vi "averaged_asap_signals.vi"(8 "error in":errorcluster, 10 "Averaging time (ms)":u32=1000, 11 "Settling time (ms)":u32=1000) -> (0 "error out":errorcluster, 1 "ASAP diagnostics":cluster{"Valid position":bool, "Message":string}, 2 "Poses":sgl[][](array[numeric]), 3 "Demodulated averaged":sgl[][](array[numeric]))   [LabVIEW 2013]
doc: "I. Description:\nThis example demonstrates how to acquire a continuous amount of data (Waveform) using the DAQ device's internal clock.\n\nII. Instructions for Running:\n1. Create an analog input voltage channel.\n2. Set the rate for the sample clock. Additionally, define the sample mode to be continuous.\n3. Call the Start VI to start the acquisition.\n4. Read the waveform data in a loop until the user hits the stop button or an error occurs.\nNote: This example reads data from one or more channels and returns an array of data. Use the Index Array function to access an individual channel of data.\n5. Call the Clear Task VI to clear the Task.\n6. Use the popup dialog box to display an error if any.\n\nIV. I/O Connections Overview:\nMake sure your signal input terminal matches the Physical Channel I/O Control. For further connection information, refer to your hardware reference manual."
uses:
  array_3d_double.ctl
  <vilib>/Platform/TimedLoop/XDataNode/timing_clust.ctl
  <vilib>/Platform/TimedLoop/XDataNode/nitl_modes.ctl
  <vilib>/Platform/TimedLoop/XDataNode/wakeup.ctl
  <vilib>/Platform/TimedLoop/XDataNode/XDataNode.xnode
  <vilib>/Platform/TimedLoop/XDataNode/XDNodeRunTimeDep.lvlib
panel:
  # "Average demodulated ASAP signals for calibration purposes.  Requires asap_monitor to be running."
  # "Lights"
  # "Channel 0"
  # "Channel 7"
  # "X"
  # "Y"
  # "Z"
  # "Match error"
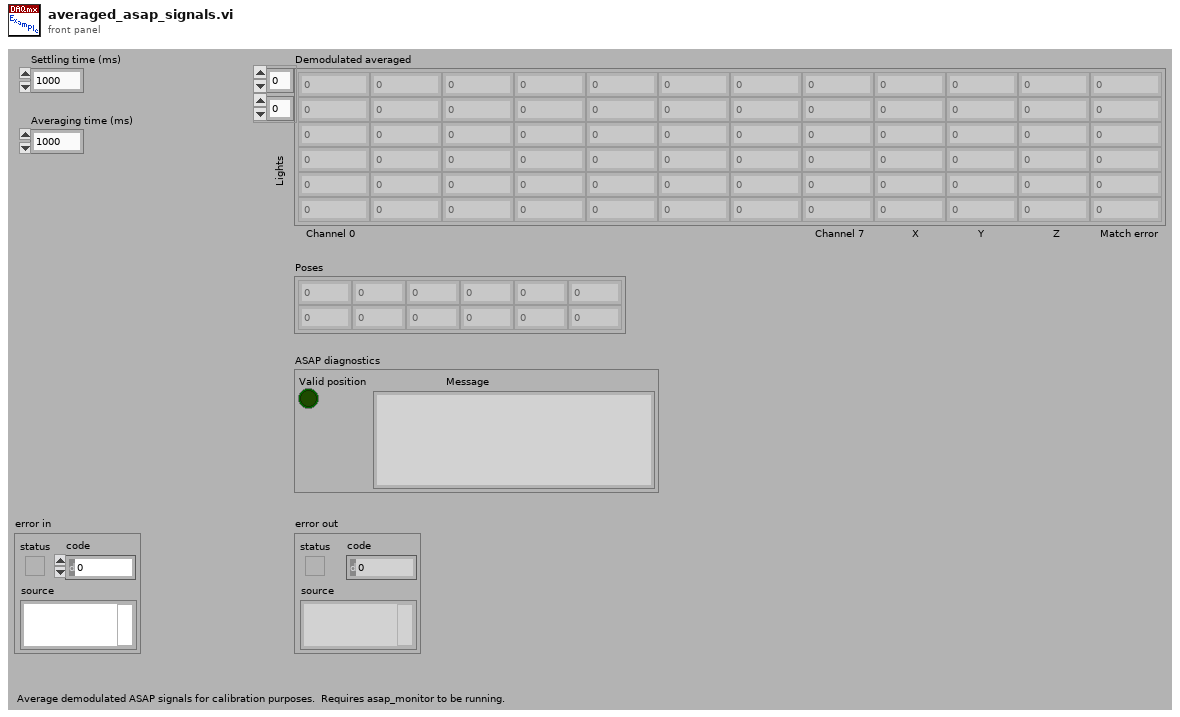
[diagram p1: front panel]
types:
  T1 = typedef "array_3d_double.ctl" = dbl[][][]
  T2 = typedef "XDNodeRunTimeDep.lvlib/timing_clust.ctl" = cluster{"Expected End [f-1]":u64, "Actual End [f-1]":u64, "Finished Late? [f-1]":bool, "Expected End [i-1]":u64, "Actual End [i-1]":u64, "Finished Late? [i-1]":bool, "Expected Start [i]":u64, "Actual Start [i]":u64, "Expected Start [f]":u64, "Actual Start [f]":u64, "Source Name":string, "Structure Name":string, "Period":i64, "Deadline":i64, "Offset":i64, "Start":i64, "Priority":i32, "Timeout":i32, "Mode":T3, "Wakeup Reason":T4, "Error":errorcluster, "Source Type":string, "Secondary Source Type":string, "Global End Time":u64, "Global Start Time":u64, "Frame Duration":u64, "Iteration Duration":u64, "Assigned CPU":i32, "I/O Scan Engine Mode":u32}
  T3 = typedef "XDNodeRunTimeDep.lvlib/nitl_modes.ctl" = enum32{"No Change", "Process missed periods, maintain original phase", "Discard missed periods, maintain original phase", "Process missed periods, ignore original phase", "Discard missed periods, ignore original phase"}
  T4 = typedef "XDNodeRunTimeDep.lvlib/wakeup.ctl" = enum32{"Normal", "Aborted", "Asynchronous wakeup", "Timing source error", "Timed loop error", "Timeout"}
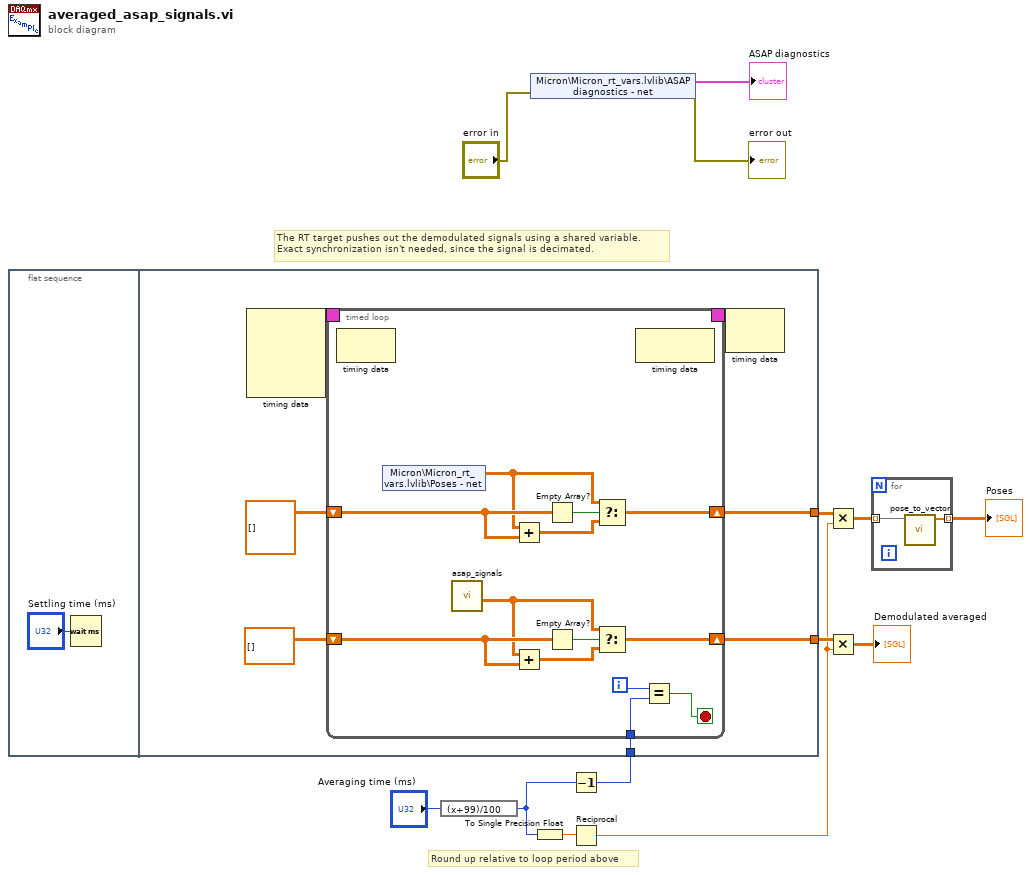
[diagram p0: block diagram]
diagram:
  # "Round up relative to loop period above"
  # "The RT target pushes out the demodulated signals using a shared variable.\nExact synchronization isn't needed, since the signal is decimated."
  n1 = flat-sequence {
    tunnel: w13 -> [w19]
    tunnel: [w18] -> w12
    tunnel: [w16] -> w4
    frame #0 {
      n2 = Wait (ms)(milliseconds to wait="Settling time (ms)") -> ()  [unwired: 1 out]
    }
    frame #1 {
      n3 = node-c288() -> (w21:T2)  [unwired: 4 in]
      n4 = timed-loop {
        timing: w21 -> [_]
        timing-out: [_] -> w20
        shift-right: [w31] -> w18
        shift-left: sgl[][] [] ("Array of Single") -> [w32]
        tunnel: w19 -> [w28]
        shift-right: [w26] -> w16
        shift-left: T1 [] ("Poses (net)") -> [w25]
        i -> [w30]
        stop <- w29 stop-if-true
        n5 = node-c288() -> ()  [unwired: 1 in, 1 out]
        n6 = shared-variable "Micron\\Micron_rt_vars.lvlib\\Poses - net"() -> (w22:T1)  [unwired: 1 in, 1 out]
        n7 = call "asap_signals.vi"() -> ("ASAP signals"=w27:sgl[][])  [unwired: 10 in, 1 out]
        n8 = Add(x=w22, y=w25) -> (x+y=w24:T1)
        n9 = Add(x=w27, y=w32) -> (x+y=w33:sgl[][])
        n10 = Empty Array?(array=w25) -> (empty?=w23:bool)
        n11 = Empty Array?(array=w32) -> (empty?=w34:bool)
        n12 = Select(t=w22, s=w23, f=w24) -> (s? t:f=w26:T1)
        n13 = Select(t=w27, s=w34, f=w33) -> (s? t:f=w31:sgl[][])
        n14 = node-c288() -> ()  [unwired: 1 in, 1 out]
        n15 = Equal?(x=w30, y=w28) -> (x = y?=w29:bool)
      }
      n16 = node-c288(w20) -> ()  [unwired: 1 out]
    }
  }
  n17 = expression code="(x+99)/100"("Averaging time (ms)") -> (w6:u32)
  n18 = shared-variable "Micron\\Micron_rt_vars.lvlib\\ASAP diagnostics - net"(error in="error in") -> (→"ASAP diagnostics":cluster{"Valid position":bool, "Message":string}, error out=→"error out":errorcluster)
  n19 = To Single Precision Float(number=w6) -> (single precision float=w11:sgl)
  n20 = Decrement(x=w6) -> (x-1=w13:u32)
  n21 = Reciprocal(x=w11) -> (1/x=w3:sgl)
  n22 = Multiply(x=w4, y=w3) -> (x*y=w2:T1)
  n23 = Multiply(x=w12, y=w3) -> (x*y=→"Demodulated averaged":sgl[][])
  n24 = for {
    tunnel: w2 -> [w40] mode=indexing
    tunnel: [w39] -> w1 mode=indexing
    n25 = call "pose_to_vector.vi"("Pose"=w40) -> ("Pose vector"=w39:dbl[])  [unwired: 10 in]
  }
  "Poses" <- w1
